vi "Day 14 Task 1.vi"() -> ()   [LabVIEW 2018]
uses:
  <userlib>/_OpenG.lib/array/array.llb/Remove Duplicates from 1D Array (String)__ogtk.vi
  <userlib>/_OpenG.lib/array/array.llb/Search 1D Array (String)__ogtk.vi
panel:
  out "Array 3":i32[](array[numeric])
  out "x-y":i32
  out "Output Array":string[](array[string])
  out "Array 2":i32[](array[numeric])
  in  "Steps":i32=4
  out "Array":string[](array[string])
  out "Numeric":i32
  out "Example Input (17)":string
  out "array":string[][](array[string])
  out "result string":string
  # "double it and -1"
  # "Template:     NNCB\nAfter step 1: NCNBCHB\nAfter step 2: NBCCNBBBCBHCB\nAfter step 3: NBBBCNCCNBBNBNBBCHBHHBCHB\nAfter step 4: NBBNBNBBCCNBCNCCNBBNBBNBBBNBBNBBCBHCBHHNHCBBCBHCB"
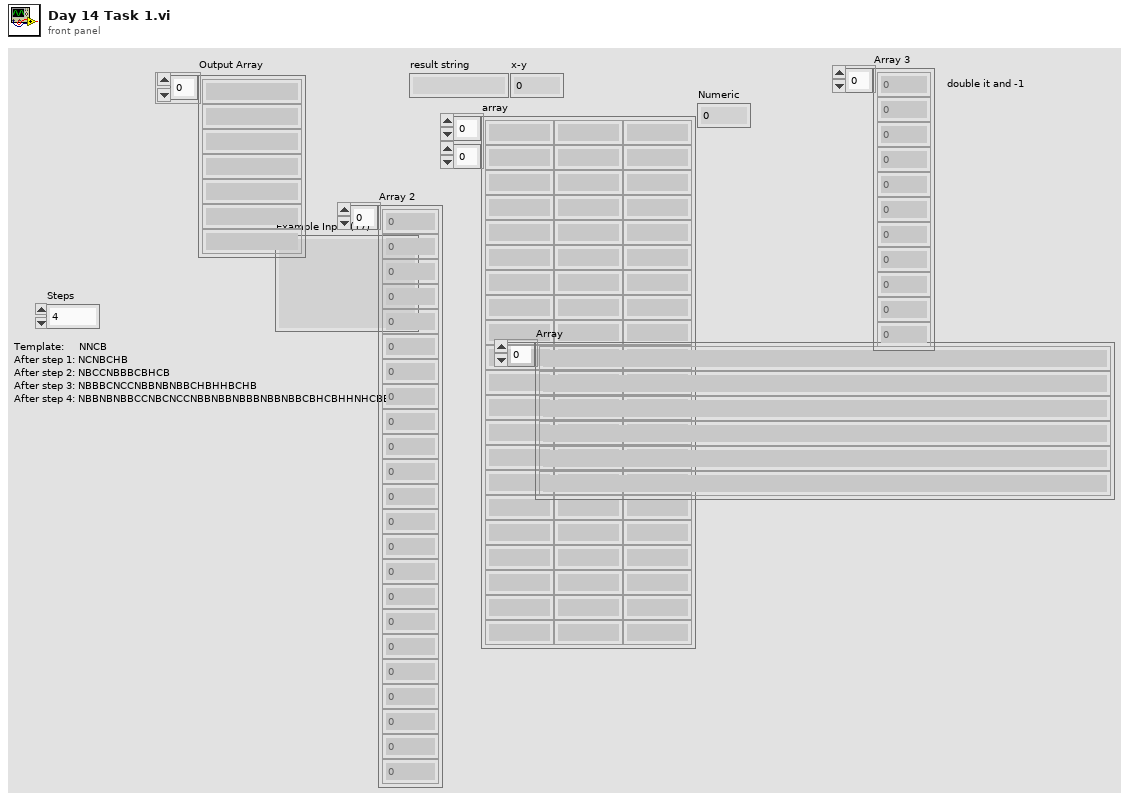
[diagram p1: front panel]
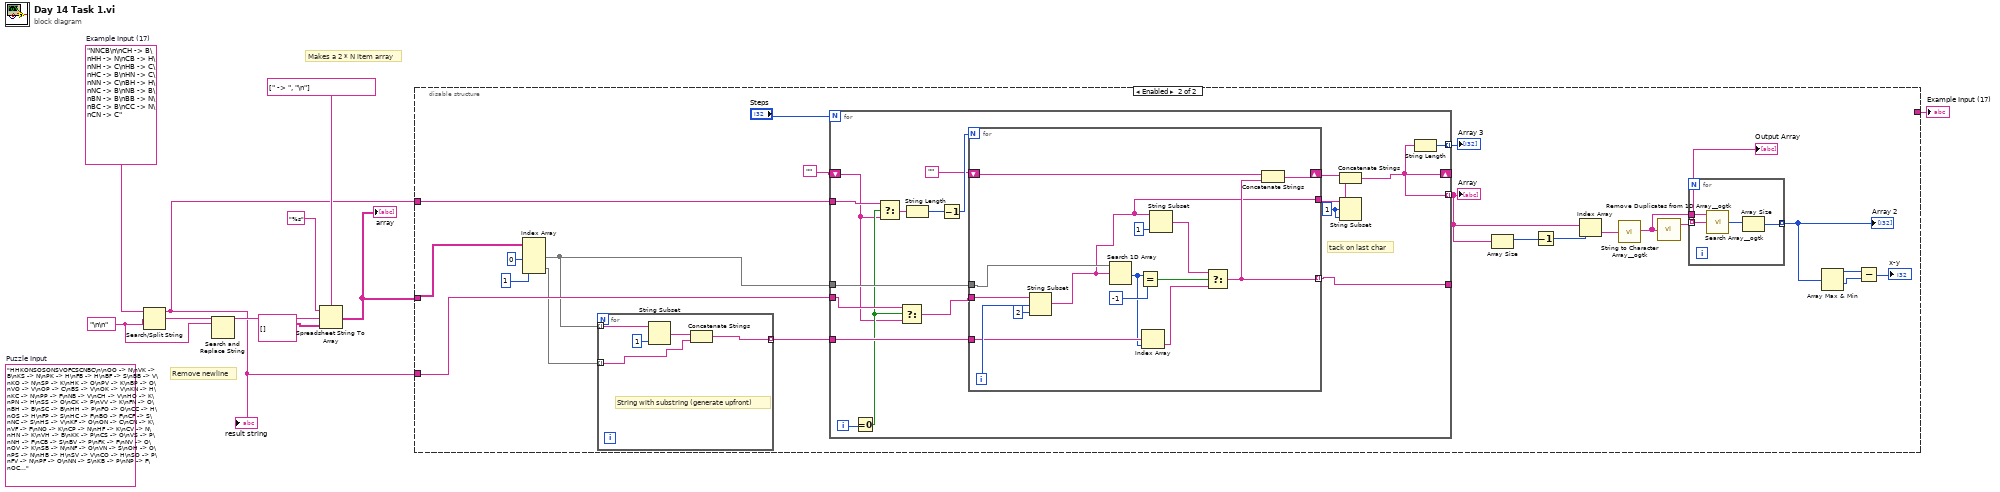
[diagram p0: block diagram]
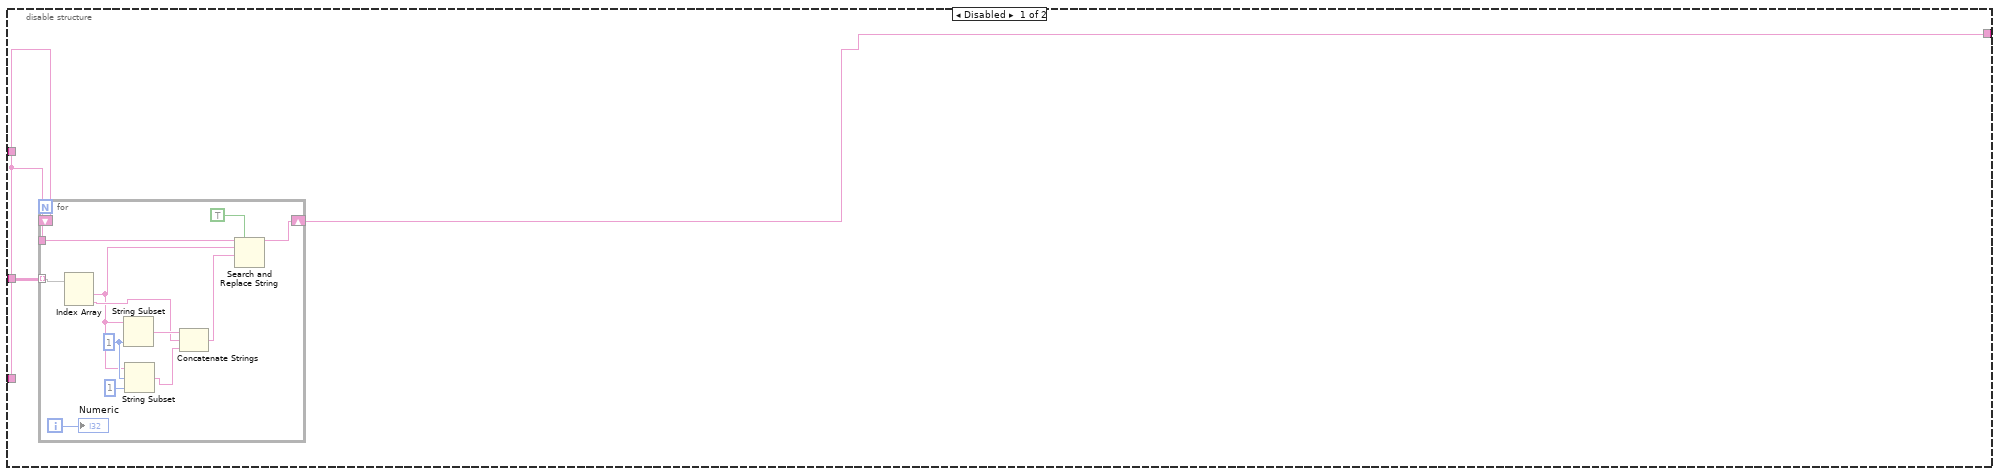
[diagram p2: hidden frame]
diagram:
  w6 = "\n\n" ("delimiter (Tab)")
  (unwired) "HHKONSOSONSVOFCSCNBC\n\nOO -> N\nVK -> B\nKS -> N\nPK -> H\nFB -> H\nBF -> S\nBB -> V\nKO -> N\nSP -> K\nHK -> O\nPV -> K\nBP -> O\nVO -> V\nOP -> C\nBS -> V\nOK -> V\nKN -> H\nKC -> N\nPP -> F\nNB -> V\nCH -> V\nHO -> K\nPN -> H\nSS -> O\nCK -> P\nVV -> K\nFN -> O\nBH -> B\nSC -> B\nHH -> P\nFO -> O\nCC -> H\nOS -> H\nFP -> S\nHC -> F\nBO -> F\nCF -> S\nNC -> S\nHS -> V\nKF -> O\nON -> C\nCN -> K\nVF -> F\nNO -> K\nCP -> N\nHF -> K\nCV -> N\nHN -> K\nVH -> B\nKK -> P\nCS -> O\nVS -> P\nNH -> F\nCB -> S\nBV -> P\nFK -> F\nNV -> O\nOV -> K\nSB -> N\nNF -> O\nVN -> S\nOH -> O\nPS -> N\nHB -> H\nSV -> V\nCO -> H\nSO -> P\nFV -> N\nPF -> O\nNN -> S\nKB -> P\nNP -> F\nOC -> S\nFS -> P\nFH -> P\nVP -> K\nBN -> O\nNS -> H\nVB -> V\nPO -> K\nKP -> N\nSN -> O\nBC -> H\nSF -> V\nPC -> O\nNK -> F\nBK -> V\nKH -> S\nSH -> S\nSK -> H\nOB -> V\nPH -> N\nPB -> C\nHV -> N\nHP -> V\nFF -> B\nOF -> P\nVC -> S\nKV -> C\nFC -> F"  # Puzzle Input
  w1 = "NNCB\n\nCH -> B\nHH -> N\nCB -> H\nNH -> C\nHB -> C\nHC -> B\nHN -> C\nNN -> C\nBH -> H\nNC -> B\nNB -> B\nBN -> B\nBB -> N\nBC -> B\nCC -> N\nCN -> C"  # Example Input (17)
  # "Remove newline"
  # "Makes a 2 * N item array"
  n1 = Search/Split String(string=w1, search string/char (-)=w6) -> (substring before match=w2:string, match + rest of string=w7:string)  [unwired: 1 in, 1 out]
  "result string" <- w2
  n2 = Search and Replace String(input string=w7, search string=w6) -> (result string=w5:string)  [unwired: 6 in, 3 out]
  n3 = Spreadsheet String To Array(delimiter (Tab)=string[] [" -> ", "\n"], format string="%s", spreadsheet string=w5, array type (2D Dbl)=string[][] []) -> (array=w4:string[][])
  "array" <- w4
  n4 = disable-structure shown="Enabled" {
    disable-tunnel: w4 -> [w13 w45]
    disable-tunnel: [w12 _] -> w3
    disable-tunnel: w2 -> [w11 w46]
    disable-tunnel: w2 -> [_ w39]
    frame Disabled {
      n5 = for {
        tunnel: w13 -> [w24] mode=indexing
        shift-right: [w25] -> w12
        shift-left: w11 -> [_]
        tunnel: w11 -> [w15]
        i -> [w14]
        w22 = 1 ("length (rest)")
        n6 = Index Array(array=w24) -> (element #1=w16:string, element #2=w19:string)  [unwired: 2 in]
        n7 = String Subset(string=w16, length (rest)=w22) -> (substring=w21:string)  [unwired: 1 in]
        n8 = String Subset(string=w16, offset (0)=w22, length (rest)=1 ("length (rest)")) -> (substring=w20:string)
        n9 = Concatenate Strings(w21, w19, w20) -> (w18:string)
        n10 = Search and Replace String(replace all?=TRUE ("replace all? (F)"), input string=w15, search string=w16, replace string=w18) -> (result string=w25:string)  [unwired: 4 in, 3 out]
        "Numeric" <- w14
      }
    }
    frame Enabled {
      n11 = Index Array(array=w45, index (col) #1=0 ("disabled index (col)"), index (col) #2=1 ("index (col)")) -> (element #1=w42:string[], element #2=w41:string[])  [unwired: 2 in]
      n12 = for {
        tunnel: w42 -> [w85] mode=indexing
        tunnel: w41 -> [w87] mode=indexing
        tunnel: [w86] -> w40 mode=indexing
        # "String with substring (generate upfront)"
        n13 = String Subset(string=w85, length (rest)=1 ("length (rest)")) -> (substring=w88:string)  [unwired: 1 in]
        n14 = Concatenate Strings(w88, w87) -> (w86:string)
      }
      n15 = for {
        N: "Steps" -> [_]
        tunnel: w46 -> [w61]
        tunnel: w42 -> [w69]
        tunnel: w40 -> [w68]
        tunnel: [w67] -> _
        tunnel: w39 -> [w62]
        shift-right: [w52] -> _
        shift-left: "" -> [w59]
        tunnel: [w52] -> w36 mode=indexing
        tunnel: [w51] -> w26 mode=indexing
        i -> [w66]
        w55 = 1 ("offset (0)")
        # "tack on last char"
        n16 = Equal To 0?(x=w66) -> (x = 0?=w60:bool)
        n17 = Select(t=w62, s=w60, f=w59) -> (s? t:f=w63:string)
        n18 = Select(t=w61, s=w60, f=w59) -> (s? t:f=w58:string)
        n19 = String Length(string=w63) -> (length=w65:i32)
        n20 = Decrement(x=w65) -> (x-1=w64:i32)
        n21 = for {
          N: w64 -> [_]
          tunnel: w58 -> [w84]
          tunnel: w69 -> [w81]
          tunnel: w68 -> [w79]
          tunnel: [w74] -> w67 mode=indexing
          shift-right: [w72] -> w57
          shift-left: "" -> [w73]
          tunnel: [w70] -> w56
          i -> [w83]
          n22 = String Subset(string=w84, offset (0)=w83, length (rest)=2 ("length (rest)")) -> (substring=w70:string)
          n23 = Search 1D Array(1D array=w81, element=w70) -> (index of element=w78:i32)  [unwired: 1 in]
          n24 = Equal?(x=w78, y=-1) -> (x = y?=w77:bool)
          n25 = Index Array(array=w79, index=w78) -> (element=w71:string)
          n26 = String Subset(string=w70, length (rest)=1 ("length (rest)")) -> (substring=w75:string)  [unwired: 1 in]
          n27 = Select(t=w75, s=w77, f=w71) -> (s? t:f=w74:string)
          n28 = Concatenate Strings(w73, w74) -> (w72:string)
        }
        n29 = String Subset(string=w56, offset (0)=w55, length (rest)=w55) -> (substring=w54:string)
        n30 = Concatenate Strings(w57, w54) -> (w52:string)
        n31 = String Length(string=w52) -> (length=w51:i32)
      }
      "Array" <- w36
      "Array 3" <- w26
      n32 = Array Size(array=w36) -> (size(s)=w31:i32)
      n33 = Decrement(x=w31) -> (x-1=w32:i32)
      n34 = Index Array(array=w36, index=w32) -> (element=w35:string)
      n35 = call <userlib>:"String to Character Array__ogtk.vi"("Input String"=w35) -> ("Character Array"=w34:string[])
      n36 = call-poly <userlib>:"Remove Duplicates from 1D Array__ogtk.vi"("Input Array"=w34) -> ("Output Array"=w33:string[])  [unwired: 1 out]
      "Output Array" <- w33
      n37 = for {
        tunnel: w34 -> [w50]
        tunnel: w33 -> [w49] mode=indexing
        tunnel: [w47] -> w30 mode=indexing
        n38 = call-poly <userlib>:"Search Array__ogtk.vi"("Array"=w50, "Element Data"=w49) -> ("Indices of Elements"=w48:i32[])  [unwired: 7 in]
        n39 = Array Size(array=w48) -> (size(s)=w47:i32)
      }
      "Array 2" <- w30
      n40 = Array Max & Min(array=w30) -> (max value=w29:i32, min value=w28:i32)  [unwired: 2 out]
      n41 = Subtract(x=w29, y=w28) -> (x-y=→"x-y":i32)
    }
  }
  "Example Input (17)" <- w3
